vi "To Serial Form.vi"(6 "Serial Version":T1, 10 "Serializer in":refnum<class "Serializer.lvclass">, 11 "String Data in":refnum<class "String Data.lvclass">) -> (0 "error out":errorcluster, 2 "Serializer out":refnum<class "Serializer.lvclass">, 3 "String Data out":refnum<class "String Data.lvclass">)   [LabVIEW 2014, in "Base Data Class.lvlib" / "String Data.lvclass"]
uses:
  String Data.lvclass
  <vilib>/NI/AQ Character Lineator/Serializer/Serializer.lvclass
  <vilib>/NI/AQ Character Lineator/Serialization Common/Serial Version.ctl
  String Data.lvclass/String Data.ctl
  <vilib>/NI/AQ Character Lineator/Serializable/Insert String.vi
  <vilib>/NI/AQ Character Lineator/Serializer/Insert String.vi
  <vilib>/NI/AQ Character Lineator/Serializer/Read Include Default Values.vi
  Data.lvclass
  <vilib>/NI/AQ Character Lineator/Serializable/Serializable.lvclass
  <vilib>/NI/AQ Character Lineator/Serialization Common/Serialization Common.lvlib
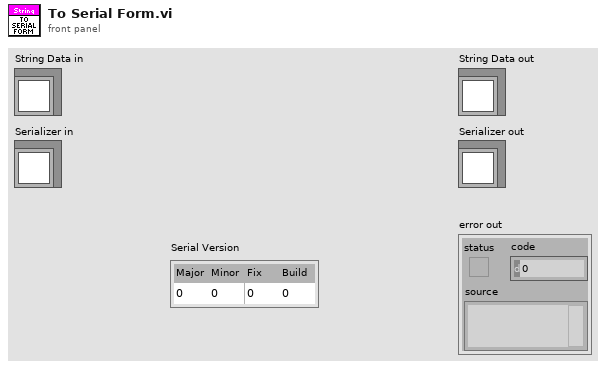
[diagram p1: front panel]
types:
  T1 = typedef "Serialization Common.lvlib/Serial Version.ctl" = cluster{"Major":u16, "Minor":u16, "Fix":u16, "Build":u16}
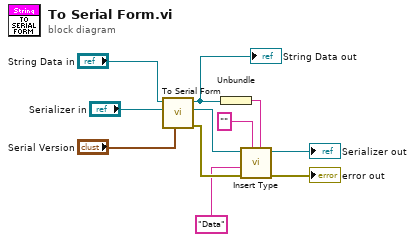
[diagram p0: block diagram]
diagram:
  n1 = call-parent "To Serial Form.vi"("Serial Version"="Serial Version", "Serializer in"="Serializer in", "Data in"="String Data in") -> ("error out"=w3:errorcluster, "Serializer out"=w2:refnum<class "Serializer.lvclass">, "Data out"=w6:refnum<class "String Data.lvclass">)  [unwired: 6 in]
  "String Data out" <- w6
  n2 = Unbundle(w6) -> (w5:string)
  n3 = call-poly <vilib>:"Insert Type.vi"("String"=w5, "Default Value"="", "error in (no error)"=w3, "Name"="Data", "Serializer in"=w2) -> ("error out"=→"error out":errorcluster, "Serializer out"=→"Serializer out":refnum<class "Serializer.lvclass">)  [unwired: 5 in]
